vi "Intellifaucet-Temp,Flow.vi"(7 "Semiphore":T1, 8 "Error In":errorcluster, 10 "TEMP,FLOW":enum8{"TEMP", "FLOW"}(ring), 11 "VISA session":refnum<visa-resource-name>="MW100") -> (0 "Error Out":errorcluster, 3 "dup VISA session":refnum<visa-resource-name>)   [LabVIEW 2009]
uses:
  ChannelSettings.ctl
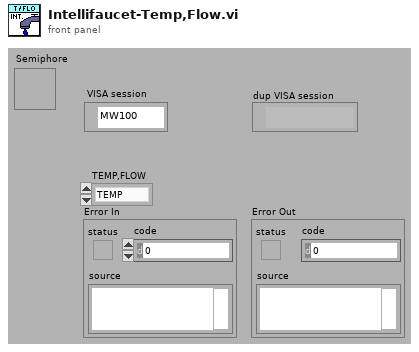
[diagram p1: front panel]
types:
  T1 = typedef "Semaphore RefNum" = refnum<k1>
  T2 = typedef "ChannelSettings.ctl" = u32
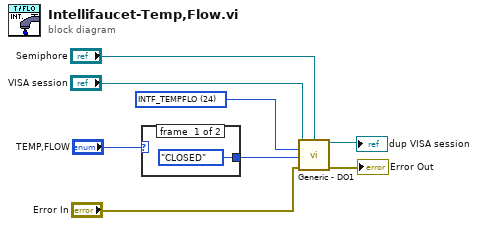
[diagram p0: block diagram]
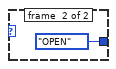
[diagram p2: hidden frame]
diagram:
  w2 = T2 24 items=["4-20_OUT", "Pres_HI1", "Pres_HI2", "Pres_LOW", "Pres_PIN", "HEATER_TOP", "HEATER_BOT", "T_Shell", "FLOWMETER", "WATT_SENSE", "WH_TICK", "Tc_1", "Tc_2", "Tc_3", "Tc_4", "Tc_5", "Tc_6", "Tc_down", "T_Shell_2", "T_Shell_3", "T_Shell_4", "RTD_IN", "RTD_OUT", "RTD_AMB", "INTF_TEMPFLO", "INTF_READY", "INTF_START", "INTF_STOP", "DRM_LOW", "DRM_HIGH", "PWR_MAIN", "VLV_DUMP", "VLV_OUT", "VLV_IN", "WATT_HOURS", "FLOW(SAMPLE)", "GALLONS", "FLOW(GPM)"] ("Channel_Enum")
  n1 = case shown="\"FLOW\"" "TEMP,FLOW" {
    tunnel: [enum8{"CLOSED", "OPEN"}."CLOSED" ("Relay Status (0:CLOSED)") enum8{"CLOSED", "OPEN"}."OPEN" ("Relay Status (0:CLOSED)")] -> w4
    frame #0 {
    }
    frame #1 {
    }
  }
  n2 = call "Generic - DO1.vi"("VISA session"="VISA session", "Semiphore"="Semiphore", "Channel_Enum"=w2, "Relay Status (0:CLOSED)"=w4, "Error In"="Error In") -> ("dup VISA session"=→"dup VISA session":refnum<visa-resource-name>, "error out"=→"Error Out":errorcluster)  [unwired: 9 in]
